vi "保存值汇总.vi"(0 "3个gap 2个贴壁 结果":bool[][](array[boolean]), 1 "3个gap 2个贴壁 亮度":dbl[][](array[numeric])) -> (4 "存档数据":dbl[](array[numeric]), 5 "数组输出":bool[](array[boolean]))   [LabVIEW 2014]
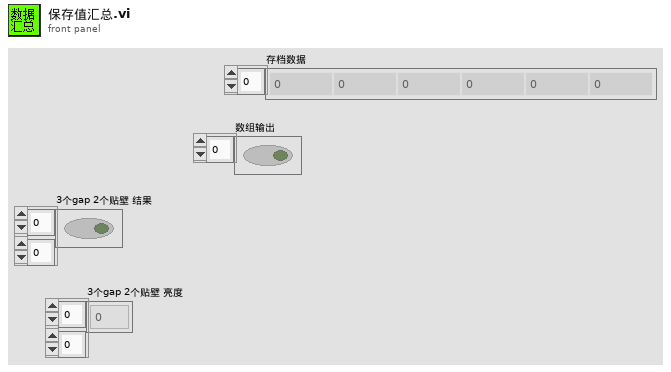
[diagram p1: front panel]
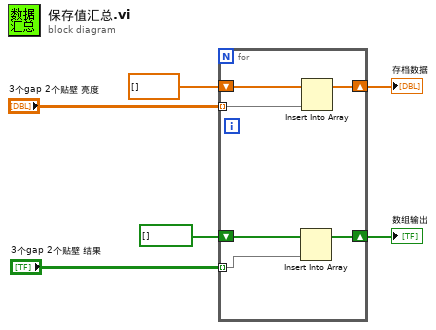
[diagram p0: block diagram]
diagram:
  n1 = for {
    shift-right: [w11] -> w3
    shift-left: dbl[] [] -> [w12]
    tunnel: "3个gap 2个贴壁 亮度" -> [w8] mode=indexing
    shift-right: [w9] -> w5
    shift-left: bool[] [] -> [w10]
    tunnel: "3个gap 2个贴壁 结果" -> [w7] mode=indexing
    n2 = Insert Into Array(array=w10, new element=w7) -> (w9:bool[])  [unwired: 1 in]
    n3 = Insert Into Array(array=w12, new element=w8) -> (w11:dbl[])  [unwired: 1 in]
  }
  "数组输出" <- w5
  "存档数据" <- w3
